vi "Advanced Cut - Add User Edit to MCLB.vi"(8 "error in (no error)":errorcluster, 9 "Edit Value":string, 10 "Coords":T1, 11 "MCListbox with Checkboxes in":refnum<class "MCListbox with Checkboxes.lvclass">) -> (0 "error out":errorcluster, 1 "Output Value":string, 3 "MCListbox with Checkboxes out":refnum<class "MCListbox with Checkboxes.lvclass">)   [LabVIEW 2016]
uses:
  UI/Listbox Class/MCListbox with Checkboxes.lvclass
  <vilib>/Utility/miscctls.llb/LVRowAndColumnTypeDef.ctl
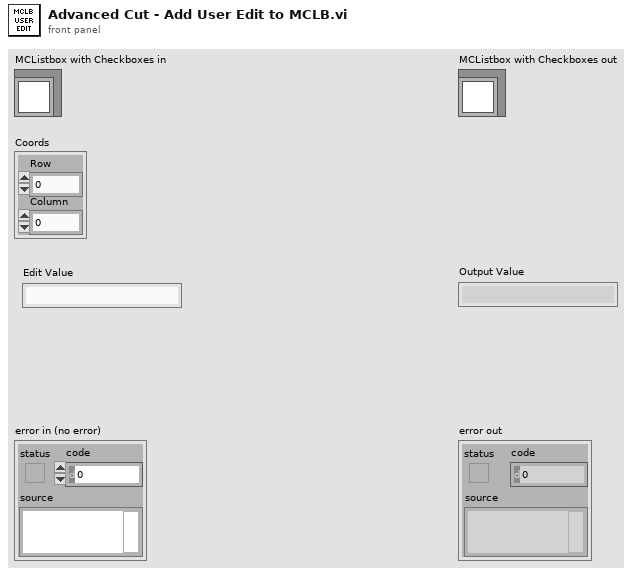
[diagram p1: front panel]
types:
  T1 = typedef "LVRowAndColumnTypeDef.ctl" = cluster{"Row":i32, "Column":i32}
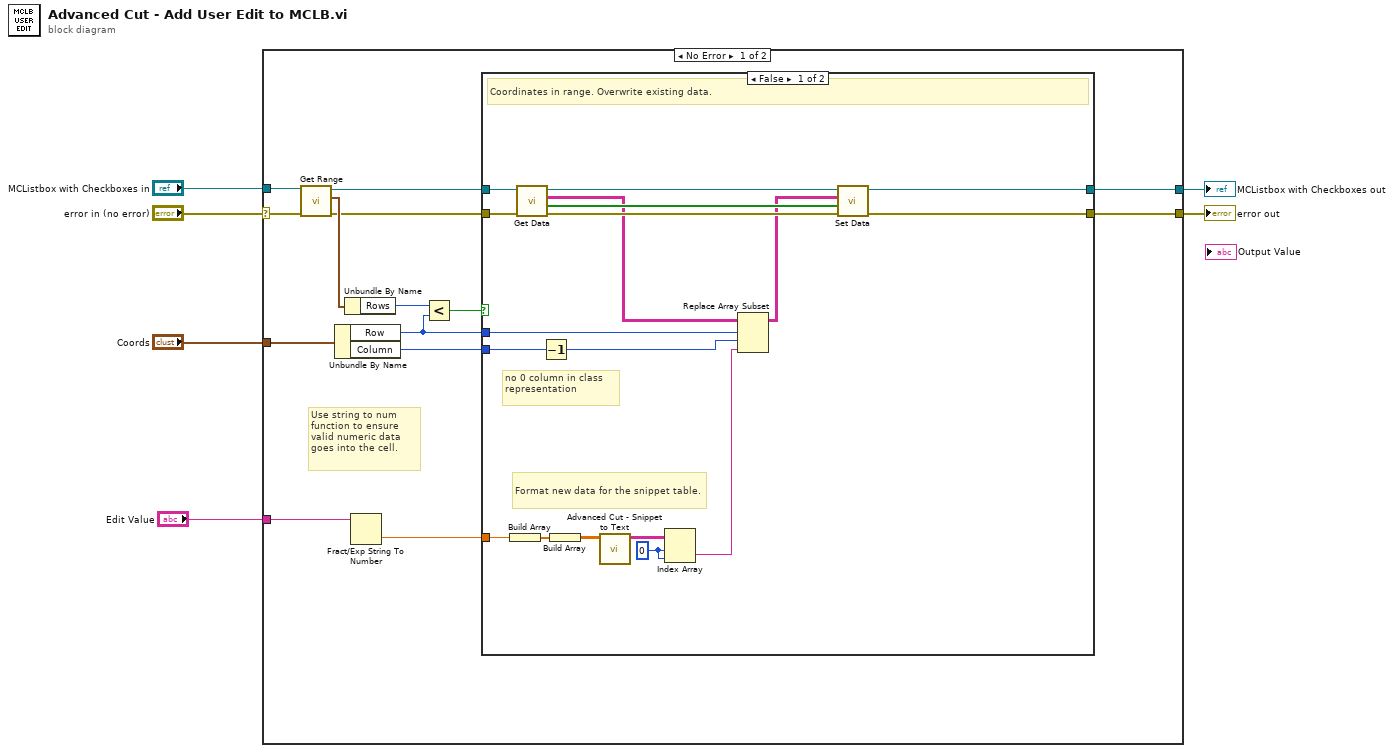
[diagram p0: block diagram]
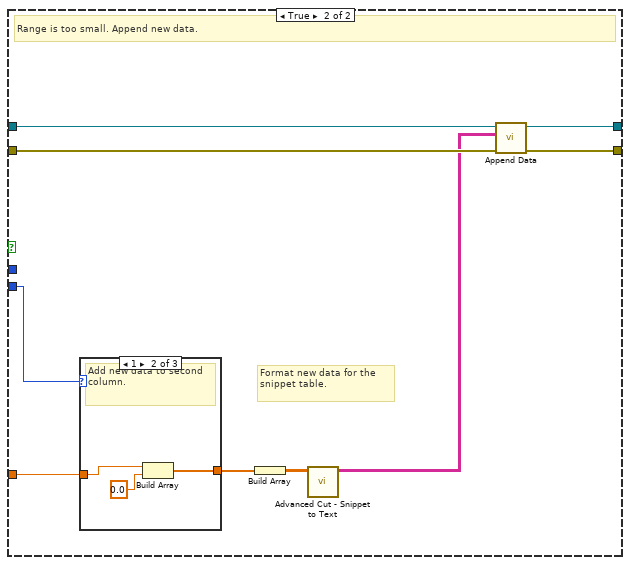
[diagram p2: hidden frame]
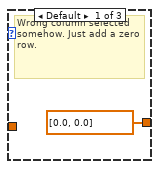
[diagram p3: hidden frame]
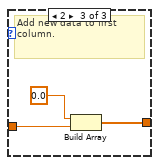
[diagram p4: hidden frame]
diagram:
  n1 = case shown="No Error" "error in (no error)" {
    selector: "error in (no error)" -> [w19 w55]
    tunnel: "MCListbox with Checkboxes in" -> [w20 w56]
    tunnel: "Coords" -> [w17 _]
    tunnel: "Edit Value" -> [w12 _]
    tunnel: [w9 w56] -> w2
    tunnel: [w8 w55] -> w1
    frame No Error {
      # "Use string to num function to ensure valid numeric data goes into the cell."
      n2 = call "Get Range.vi"("error in (no error)"=w19, "MCListbox with Checkboxes in"=w20) -> ("error out"=w13:errorcluster, "Range"=w18:cluster{"Rows":i32, "Columns":i32}, "MCListbox with Checkboxes out"=w14:refnum<class "MCListbox with Checkboxes.lvclass">)  [unwired: 7 in]
      n3 = Unbundle By Name(w17) -> ("Row"=w10:i32, "Column"=w7:i32)
      n4 = Unbundle By Name(w18) -> ("Rows"=w16:i32)
      n5 = Fract/Exp String To Number(string=w12) -> (number=w11:dbl)  [unwired: 3 in, 1 out]
      n6 = Less?(x=w16, y=w10) -> (x < y?=w15:bool)
      n7 = case shown="False" w15 {
        tunnel: w14 -> [w38 w47]
        tunnel: w13 -> [w37 w46]
        tunnel: w11 -> [w28 w45]
        tunnel: w7 -> [w29 w44]
        tunnel: w10 -> [w30 _]
        tunnel: [w34 w40] -> w9
        tunnel: [w33 w39] -> w8
        frame False {
          w24 = 0 ("index (row)")
          # "no 0 column in class representation"
          # "Format new data for the snippet table."
          # "Coordinates in range. Overwrite existing data."
          n8 = Build Array(w28) -> (w27:dbl[])
          n9 = call "Get Data.vi"("error in (no error)"=w37, "MCListbox with Checkboxes in"=w38) -> ("error out"=w35:errorcluster, "Check Data"=w32:bool[], "Cell Data"=w31:string[][], "MCListbox with Checkboxes out"=w36:refnum<class "MCListbox with Checkboxes.lvclass">)  [unwired: 6 in]
          n10 = Decrement(x=w29) -> (x-1=w21:i32)
          n11 = Build Array(w27) -> (w26:dbl[][])
          n12 = call "Advanced Cut - Snippet to Text.vi"("Numeric Snippets"=w26) -> ("String Snippets"=w25:string[][])  [unwired: 9 in, 1 out]
          n13 = Index Array(array=w25, index (row)=w24, index (col)=w24) -> (element=w23:string)
          n14 = Replace Array Subset(array=w31, new element=w23, index (row)=w30, index (col)=w21) -> (w22:string[][])
          n15 = call "Set Data.vi"("error in (no error)"=w35, "Check Data"=w32, "Cell Data"=w22, "MCListbox with Checkboxes in"=w36) -> ("error out"=w33:errorcluster, "MCListbox with Checkboxes out"=w34:refnum<class "MCListbox with Checkboxes.lvclass">)  [unwired: 6 in]
        }
        frame True {
          # "Format new data for the snippet table."
          # "Range is too small. Append new data."
          n16 = case shown="1" w44 {
            tunnel: w45 -> [_ w51 w53]
            tunnel: [dbl[] [0.0, 0.0] w50 w52] -> w43
            frame Default {
              # "Wrong column selected somehow. Just add a zero row."
            }
            frame 1 {
              # "Add new data to second column."
              n17 = Build Array(w51, 0.0 ("element")) -> (w50:dbl[])
            }
            frame 2 {
              # "Add new data to first column."
              n18 = Build Array(0.0, w53) -> (w52:dbl[])
            }
          }
          n19 = Build Array(w43) -> (w42:dbl[][])
          n20 = call "Advanced Cut - Snippet to Text.vi"("Numeric Snippets"=w42) -> ("String Snippets"=w41:string[][])  [unwired: 9 in, 1 out]
          n21 = call "Append Data.vi"("error in (no error)"=w46, "Cell Data"=w41, "MCListbox with Checkboxes in"=w47) -> ("error out"=w39:errorcluster, "MCListbox with Checkboxes out"=w40:refnum<class "MCListbox with Checkboxes.lvclass">)  [unwired: 7 in]
        }
      }
    }
    frame Error {
    }
  }
  "MCListbox with Checkboxes out" <- w2
  "error out" <- w1
